vi "Destroy.vi"(0 "reference in":refnum<class "Tester.lvclass">, 5 "error in (no error)":errorcluster) -> (14 "reference out":refnum<class "Tester.lvclass">, 19 "error out":errorcluster)   [LabVIEW 2018, in "Tester.lvclass"]
uses:
  Tester.lvclass
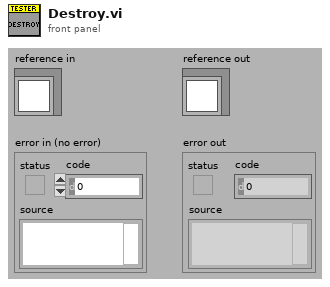
[diagram p1: front panel]
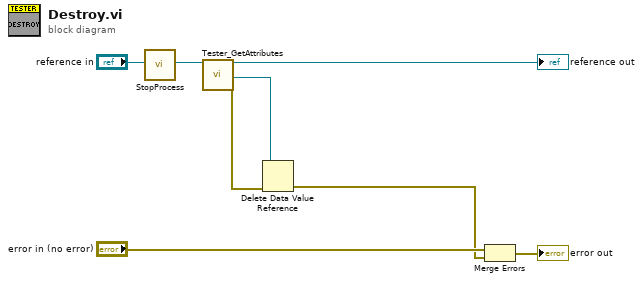
[diagram p0: block diagram]
diagram:
  n1 = call "StopProcess.vi"("reference in"="reference in") -> ("reference out"=w1:refnum<class "Tester.lvclass">)  [unwired: 17 in, 1 out]
  n2 = call "Tester_GetAttributes.vi"("reference in"=w1) -> ("reference out"=→"reference out":refnum<class "Tester.lvclass">, "DataRef"=w5:refnum<data-value>, "error out"=w6:errorcluster)  [unwired: 15 in, 1 out]
  n3 = Delete Data Value Reference(data value reference=w5, error in=w6) -> (error out=w3:errorcluster)  [unwired: 1 out]
  n4 = Merge Errors("error in (no error)", w3) -> (→"error out":errorcluster)
